vi "unscale lecroy waveform.vi"(8 "Error in":errorcluster, 11 "Waveforms":waveform(dbl)[](graph)) -> (0 "Error out":errorcluster, 2 "GEECS waveforms info":T1(array[cluster]), 3 "scope traces":i16[][](array[numeric]))   [LabVIEW 2020, in "PicoscopeV2.lvclass"]
uses:
  PicoscopeV2.lvclass
  TektronixDPOSimple/TektronixDPOSimple.lvclass
panel:
  out "Waveform Data 3":waveform(dbl)[](graph)
  out "Waveform Data 2":waveform(dbl)[](graph)
  out "WF info out":T2
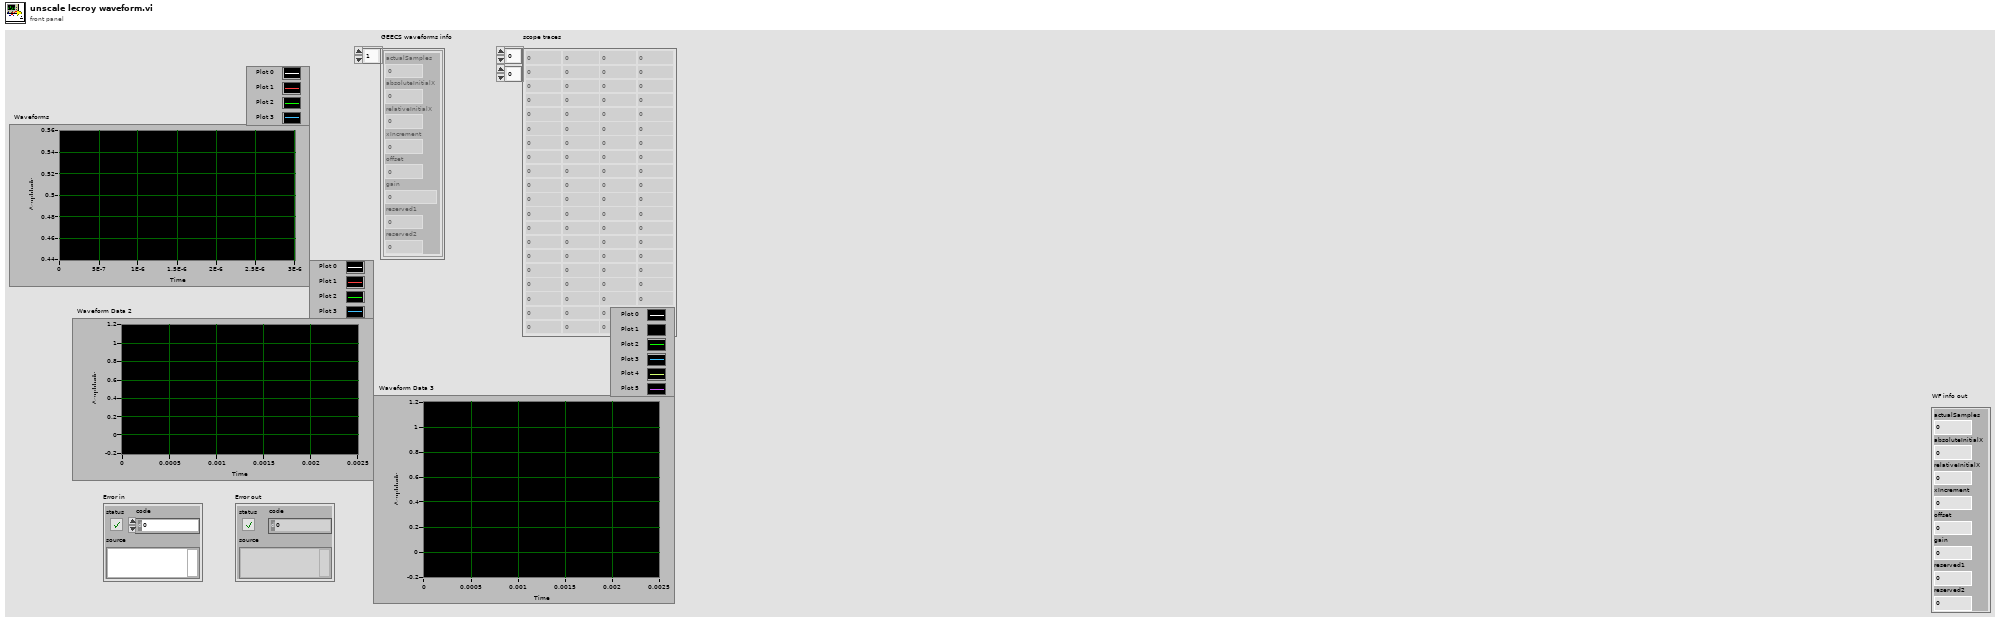
[diagram p1: front panel]
types:
  T1 = cluster{"actualSamples":i32, "absoluteInitialX":dbl, "relativeInitialX":dbl, "xIncrement":dbl, "offset":dbl, "gain":dbl, "reserved1":dbl, "reserved2":dbl}[]
  T2 = cluster{"actualSamples":i32, "absoluteInitialX":dbl, "relativeInitialX":dbl, "xIncrement":dbl, "offset":dbl, "gain":dbl, "reserved1":dbl, "reserved2":dbl}
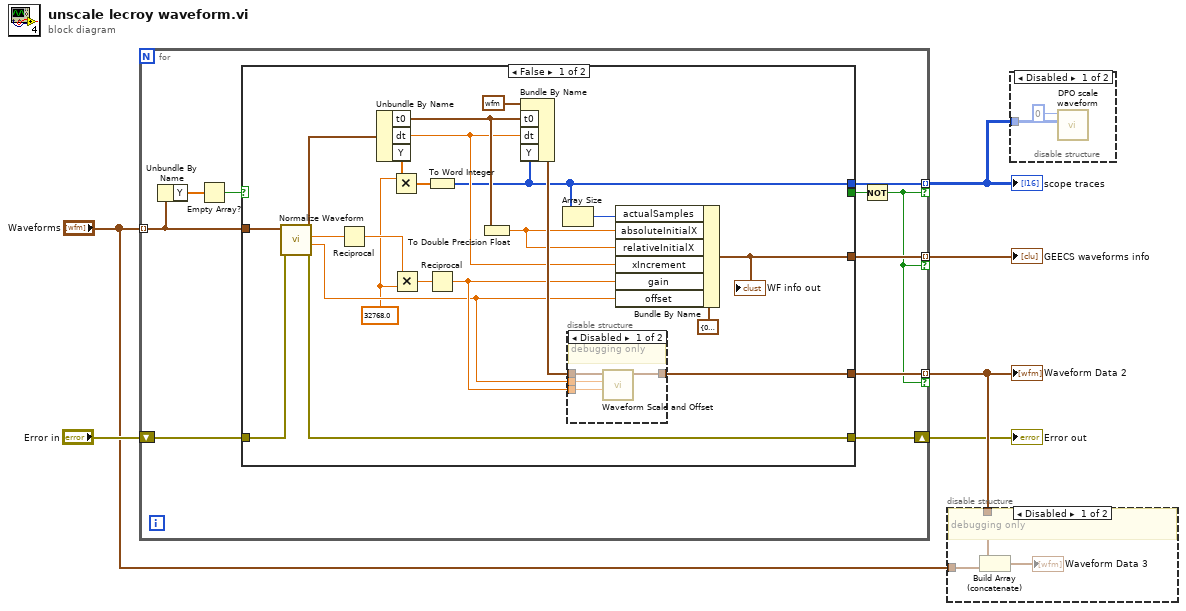
[diagram p0: block diagram]
diagram:
  n1 = for {
    tunnel: "Waveforms" -> [w13] mode=indexing
    tunnel: [w16] -> w5 mode=indexing if=w7
    tunnel: [w10] -> w6 mode=indexing if=w7
    tunnel: [w15] -> w3 mode=indexing if=w7
    shift-right: [w11] -> w2
    shift-left: "Error in" -> [w14]
    n2 = Unbundle By Name(w13) -> ("Y"=w12:dbl[])
    n3 = Empty Array?(array=w12) -> (empty?=w9:bool)
    n4 = case shown="False" w9 {
      selector: w9 -> [_ w43]
      tunnel: [w32 _] -> w16
      tunnel: [w26 _] -> w15
      tunnel: w14 -> [w20 w44]
      tunnel: w13 -> [w19 _]
      tunnel: [w18 w44] -> w11
      tunnel: [w17 _] -> w10
      tunnel: [_ w43] -> w8
      frame False {
        w23 = 32768.0
        n5 = call <vilib>:"Normalize Waveform.vi"("error in (no error)"=w20, "waveform in"=w19) -> ("error out"=w18:errorcluster, "offset"=w24:dbl, "scale"=w22:dbl, "normalized waveform"=w21:waveform(dbl))  [unwired: 6 in]
        n6 = Reciprocal(x=w22) -> (1/x=w25:dbl)
        n7 = Unbundle By Name(w21) -> ("t0"=w30:timestamp, "dt"=w29:dbl, "Y"=w37:dbl[])
        n8 = Multiply(x=w23, y=w37) -> (x*y=w36:dbl[])
        n9 = Multiply(x=w25, y=w23) -> (x*y=w28:dbl)
        n10 = To Word Integer(number=w36) -> (16bit integer=w17:i16[])
        n11 = Reciprocal(x=w28) -> (1/x=w27:dbl)
        n12 = To Double Precision Float(number=w30) -> (double precision float=w31:dbl)
        n13 = Bundle By Name(cluster=waveform(i16) {"t0"=timestamp(0 s since 1904-01-01), "dt"=1.0, "Y"=[]} ("waveform"), "t0"=w30, "dt"=w29, "Y"=w17) -> (w38:waveform(i16))
        n14 = Array Size(array=w17) -> (size(s)=w33:i32)
        n15 = disable-structure shown="Disabled" {
          disable-tunnel: w27 -> [w42 _]
          disable-tunnel: w38 -> [w41 _]
          disable-tunnel: [w40 _] -> w26
          disable-tunnel: w24 -> [w39 _]
          frame Disabled {
            # "debugging only"
            n16 = call <vilib>:"Waveform Scale and Offset.vi"("scale"=w42, "offset"=w39, "waveform in"=w41) -> ("waveform out"=w40:waveform(dbl))  [unwired: 7 in, 1 out]
          }
          frame Enabled {
          }
        }
        n17 = Bundle By Name(cluster=T2 {"actualSamples"=0, "absoluteInitialX"=0.0, "relativeInitialX"=0.0, "xIncrement"=0.0, "offset"=0.0, "gain"=0.0, "reserved1"=0.0, "reserved2"=0.0} ("waveform info"), "actualSamples"=w33, "absoluteInitialX"=w31, "relativeInitialX"=w31, "xIncrement"=w29, "gain"=w27, "offset"=w24) -> (w32:T2)
        "WF info out" <- w32
      }
      frame True {
      }
    }
    n18 = Not(x=w8) -> (.not. x?=w7:bool)
  }
  "GEECS waveforms info" <- w5
  "scope traces" <- w6
  "Waveform Data 2" <- w3
  "Error out" <- w2
  n19 = disable-structure shown="Disabled" {
    disable-tunnel: w3 -> [w47 _]
    disable-tunnel: "Waveforms" -> [w45 _]
    frame Disabled {
      # "debugging only"
      n20 = Build Array (concatenate)(w47, w45) -> (→"Waveform Data 3":waveform(dbl)[])
    }
    frame Enabled {
    }
  }
  n21 = disable-structure shown="Disabled" {
    disable-tunnel: w6 -> [w48 _]
    frame Disabled {
      n22 = call "DPO scale waveform.vi"("I16 in"=w48, "Number of waveforms"=0) -> ()  [unwired: 6 in, 4 out]
    }
    frame Enabled {
    }
  }
